vi "Configure Trigger Source.vi"(8 "error in (no error)":errorcluster, 9 "Source (Software)":string(combo)="BUS", 11 "VISA resource name":refnum<visa-resource-name>) -> (0 "error out":errorcluster, 3 "VISA resource name out":refnum<visa-resource-name>)   [LabVIEW 2018, in "Agilent E364X Series.lvlib"]
doc: "Configures the trigger source the power supply waits for before changing the output signal. When the power supply receives a trigger signal on the source you specify, it changes its current limit and voltage level to the values of the pending trigger current and voltage levels."
uses:
  Agilent E364X Series.lvlib
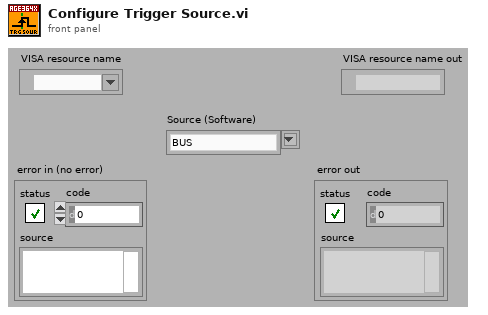
[diagram p1: front panel]
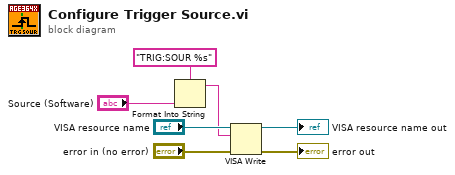
[diagram p0: block diagram]
diagram:
  n1 = Format Into String(format string="TRIG:SOUR %s", "Source (Software)") -> (resulting string=w3:string)  [unwired: 2 in, 1 out]
  n2 = VISA Write(VISA resource name="VISA resource name", write buffer=w3, error in (no error)="error in (no error)") -> (VISA resource name out=→"VISA resource name out":refnum<visa-resource-name>, error out=→"error out":errorcluster)  [unwired: 1 out]
